vi "ProcessInput.vi"(8 "Error In (no error)":errorcluster, 10 "TeleopData":T1) -> (0 "Error Out":errorcluster)   [LabVIEW 2013]
doc: "Takes data from teleop and determines what instructions, if any, need to be enqueued."
uses:
  TeleopData.ctl
  Robot Global Data.vi
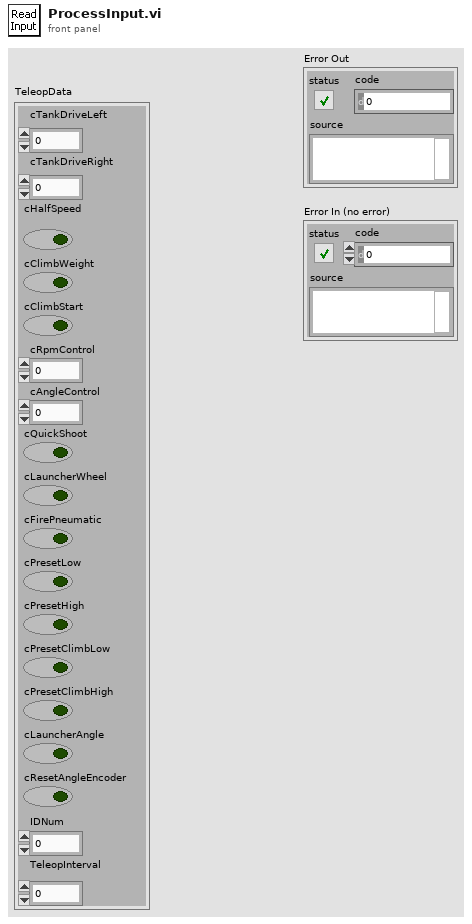
[diagram p1: front panel]
types:
  T1 = typedef "TeleopData.ctl" = cluster{"cTankDriveLeft":dbl, "cTankDriveRight":dbl, "cHalfSpeed":bool, "cClimbWeight":bool, "cClimbStart":bool, "cRpmControl":dbl, "cAngleControl":dbl, "cQuickShoot":bool, "cLauncherWheel":bool, "cFirePneumatic":bool, "cPresetLow":bool, "cPresetHigh":bool, "cPresetClimbLow":bool, "cPresetClimbHigh":bool, "cLauncherAngle":bool, "cResetAngleEncoder":bool, "IDNum":i32, "TeleopInterval":i32}
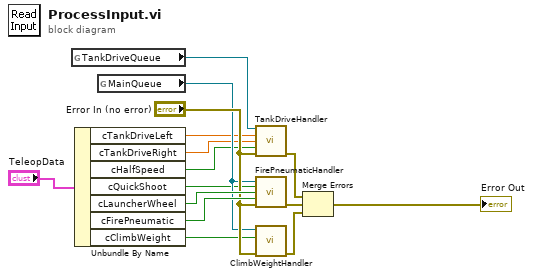
[diagram p0: block diagram]
diagram:
  n1 = global read "Robot Global Data.vi" "TankDriveQueue"() -> (w11:refnum<queue>)
  n2 = Unbundle By Name("TeleopData") -> ("cTankDriveLeft"=w2:dbl, "cTankDriveRight"=w3:dbl, "cHalfSpeed"=w1:bool, "cQuickShoot"=w4:bool, "cLauncherWheel"=w9:bool, "cFirePneumatic"=w10:bool, "cClimbWeight"=w5:bool)
  n3 = global read "Robot Global Data.vi" "MainQueue"() -> (w7:refnum<queue>)
  n4 = call "TankDriveHandler.vi"("TankDrive Queue"=w11, "Left Motor Value"=w2, "Right Motor Value"=w3, "HalfSpeed (F)"=w1, "Error In (no error)"="Error In (no error)") -> ("Error Out"=w14:errorcluster)  [unwired: 10 in]
  n5 = call "FirePneumaticHandler.vi"("MainQueue"=w7, "cQuickShoot"=w4, "cLauncherWheel"=w9, "cFirePneumatic"=w10, "error in (no error)"="Error In (no error)") -> ("error out"=w13:errorcluster)  [unwired: 10 in]
  n6 = call "ClimbWeightHandler.vi"("error in (no error)"="Error In (no error)", "cClimbWeight"=w5, "MainQueue"=w7) -> ("error out"=w6:errorcluster)  [unwired: 8 in]
  n7 = Merge Errors(w14, w13, w6) -> (→"Error Out":errorcluster)
